vi "Write.vi"(8 "error in (no error)":errorcluster, 9 "Value":variant, 10 "Symbol Name":string, 11 "TwinCAT ADS in":refnum<class "TwinCAT ADS.lvclass">) -> (0 "error out":errorcluster, 3 "TwinCAT ADS out":refnum<class "TwinCAT ADS.lvclass">)   [LabVIEW 2018, in "TwinCAT ADS.lvclass"]
uses:
  TwinCAT ADS.lvclass
  TwinCAT ADS.lvclass/TwinCAT ADS.ctl
  TwinCAT.Ads
  Get From Symbol Map.vi
  Get From Symbol Map Daemon.vi
  Get Symbol Map.vi
  Format String.vi
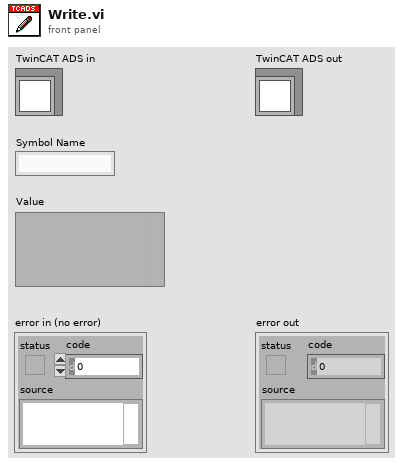
[diagram p1: front panel]
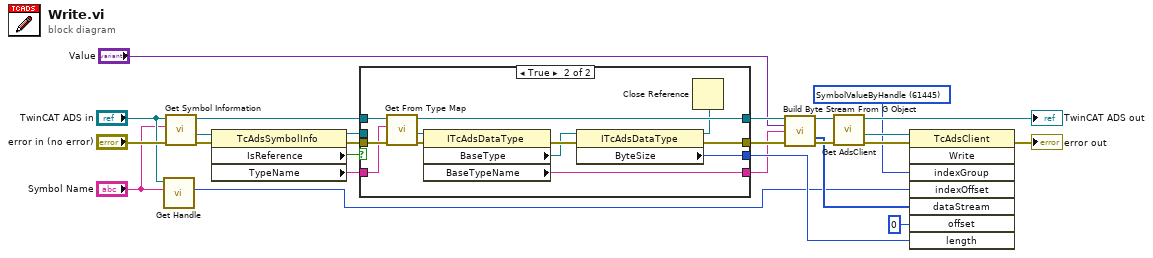
[diagram p0: block diagram]
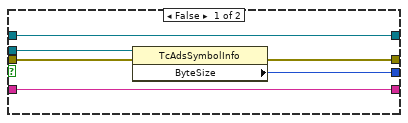
[diagram p2: hidden frame]
diagram:
  w16 = u32 61445 items=["PlcRWIB"=16384, "PlcRWOB"=16400, "PlcRWMB"=16416, "PlcRWRB"=16432, "PlcRWDB"=16448, "SymbolTable"=61440, "SymbolName"=61441, "SymbolValue"=61442, "SymbolHandleByName"=61443, "SymbolValueByName"=61444, "SymbolValueByHandle"=61445, "SymbolReleaseHandle"=61446, "SymbolInfoByName"=61447, "SymbolVersion"=61448, "SymbolInfoByNameEx"=61449, "SymbolDownload"=61450, "SymbolUpload"=61451, "SymbolUploadInfo"=61452, "SymbolNote"=61456, "IOImageRWIB"=61472, "IOImageRWIX"=61473, "IOImageRWOB"=61488, "IOImageRWOX"=61489, "IOImageClearI"=61504, "IOImageClearO"=61520, "SumCommandRead"=61568, "SumCommandWrite"=61569, "SumCommandReadWrite"=61570, "SumCommandReadEx"=61571, "SumCommandReadEx2"=61572, "SumCommandAddDevNote"=61573, "SumCommandDelDevNote"=61574, "DeviceData"=61696] ("SumCommandRead")
  n1 = call "Get Handle.vi"("Symbol Name"="Symbol Name", "TwinCAT ADS in"="TwinCAT ADS in") -> ("Handle"=w1:i32)  [unwired: 7 in, 2 out]
  n2 = call "Get Symbol Information.vi"("error in (no error)"="error in (no error)", "Symbol Name"="Symbol Name", "TwinCAT ADS in"="TwinCAT ADS in") -> ("error out"=w12:errorcluster, ".NET Symbol Information"=w11:refnum<k24>, "TwinCAT ADS out"=w9:refnum<class "TwinCAT ADS.lvclass">)  [unwired: 6 in]
  n3 = property class="TcAdsSymbolInfo"(reference=w11, error in=w12) -> (reference out=w7:refnum<k24>, error out=w8:errorcluster, "IsReference"=w6:bool, "TypeName"=w5:string)
  n4 = case shown="True" w6 {
    tunnel: w8 -> [w31 w43]
    tunnel: [w27 w39] -> w25
    tunnel: w5 -> [w26 w40]
    tunnel: [w26 w32] -> w2
    tunnel: [w28 w36] -> w3
    tunnel: [w29 w34] -> w4
    tunnel: w7 -> [w30 _]
    tunnel: w9 -> [w27 w33]
    frame False {
      n5 = property class="TcAdsSymbolInfo"(reference=w30, error in=w31) -> (error out=w29:errorcluster, "ByteSize"=w28:i32)  [unwired: 1 out]
    }
    frame True {
      n6 = call "Get From Type Map.vi"("error in (no error)"=w43, "Type Name"=w40, "TwinCAT ADS in"=w33) -> ("error out"=w42:errorcluster, ".NET AdsDataType"=w41:refnum<k24>, "TwinCAT ADS out"=w39:refnum<class "TwinCAT ADS.lvclass">)  [unwired: 6 in]
      n7 = property class="ITcAdsDataType"(reference=w41, error in=w42) -> (error out=w38:errorcluster, "BaseType"=w37:refnum<k24>, "BaseTypeName"=w32:string)  [unwired: 1 out]
      n8 = property class="ITcAdsDataType"(reference=w37, error in=w38) -> (reference out=w35:refnum<k24>, error out=w34:errorcluster, "ByteSize"=w36:i32)
      n9 = Close Reference(reference=w35) -> ()  [unwired: 1 in, 1 out]
    }
  }
  n10 = call "Build Byte Stream From G Object.vi"("TwinCAT ADS in"=w25, "Value"="Value", "Type Name"=w2, "error in (no error)"=w4) -> ("TwinCAT ADS out"=w19:refnum<class "TwinCAT ADS.lvclass">, "Byte Stream out"=w10:u8[], "error out"=w20:errorcluster)  [unwired: 9 in]
  n11 = call "Get AdsClient.vi"("error in (no error)"=w20, "TwinCAT ADS in"=w19) -> ("error out"=w24:errorcluster, ".NET TcAdsClient"=w23:refnum<k24>, "TwinCAT ADS out"=→"TwinCAT ADS out":refnum<class "TwinCAT ADS.lvclass">)  [unwired: 7 in]
  n12 = invoke class="TcAdsClient" method="Write"(reference=w23, error in=w24, "indexGroup"=w16, "indexOffset"=w1, "dataStream"=w10, "offset"=0, "length"=w3) -> (error out=→"error out":errorcluster)  [unwired: 1 in, 7 out]
